vi "lolipoop.vi"() -> ()   [LabVIEW 2018]
panel:
  in  "Dial":dbl(knob) scale=0.0..10.0
  in  "Numeric":dbl
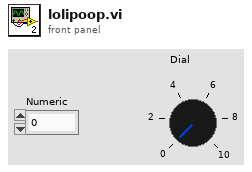
[diagram p1: front panel]
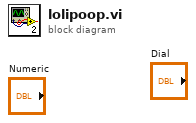
[diagram p0: block diagram]
diagram:
